vi "LoadControlPanel.vi"(8 "error in (no error)":errorcluster, 10 "Actor In":refnum<class "Actor.lvclass">, 11 "Laser_Oxxius in":refnum<class "Laser_Oxxius.lvclass">) -> (0 "error out":errorcluster, 3 "Laser_Oxxius out":refnum<class "Laser_Oxxius.lvclass">)   [LabVIEW 2020, in "Laser_Oxxius.lvlib" / "Laser_Oxxius.lvclass"]
uses:
  Laser_Oxxius.lvclass
  ViewController/OxxiusLaserController/OxxiusLaserController.lvclass
  Hardware Abstraction Layer/Component/Laser/Laser/Laser.lvclass
  C:/Program Files/National Instruments/LabVIEW 2020/vi.lib/ActorFramework/Actor/Actor.lvclass
  <vilib>/ActorFramework/Actor/Actor.lvclass
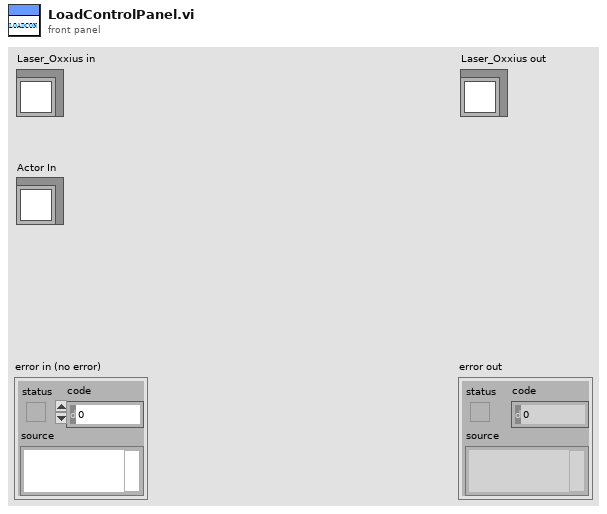
[diagram p1: front panel]
types:
  T1 = typedef "DataListener.lvclass/DataExchange.ctl" = cluster{"Source":string, "Destination":string, "Description":string, "value":variant}
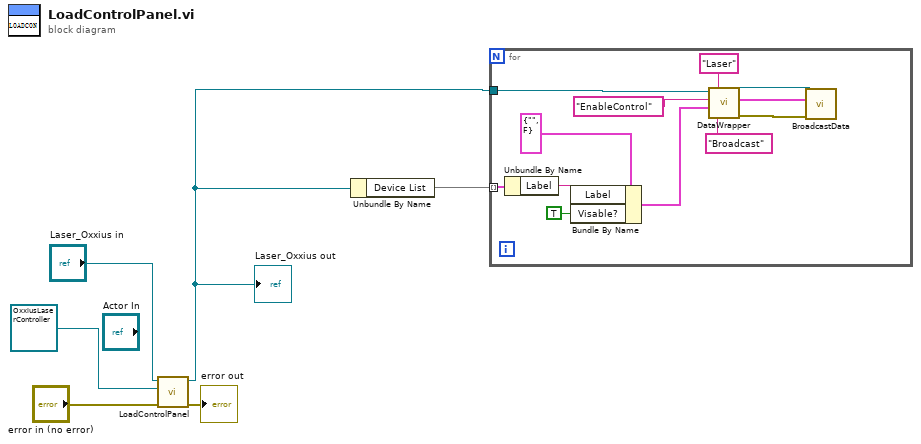
[diagram p0: block diagram]
diagram:
  n1 = call-parent "LoadControlPanel.vi"("error in (no error)"="error in (no error)", "Actor In"=refnum<class "OxxiusLaserController.lvclass"> refnum ("OxxiusLaserController.lvlib:OxxiusLaserController.lvclass"), "GRMActor in"="Laser_Oxxius in") -> ("error out"=→"error out":errorcluster, "GRMActor out"=w1:refnum<class "Laser_Oxxius.lvclass">)  [unwired: 7 in]
  "Laser_Oxxius out" <- w1
  n2 = Unbundle By Name(w1) -> ("Device List"=w2:map{string, refnum<k24>})
  n3 = for {
    tunnel: w2 -> [w18] mode=indexing
    tunnel: w1 -> [w14]
    n4 = Unbundle By Name(w18) -> ("Label"=w16:string)
    n5 = Bundle By Name(cluster=cluster{"Label":string, "Visable?":bool} {"Label"="", "Visable?"=FALSE} ("event data"), "Label"=w16, "Visable?"=TRUE) -> (w10:cluster{"Label":string, "Visable?":bool})
    n6 = call-dynamic "DataWrapper.vi"("Destination"="Broadcast" ("Type"), "Source"="Laser", "value"=w10, "Description"="EnableControl" ("Target"), "GRMActor in"=w14) -> ("error out"=w7:errorcluster, "DataExchange"=w8:T1, "GRMActor out"=w9:refnum<class "Laser_Oxxius.lvclass">)  [unwired: 4 in]
    n7 = call-dynamic "BroadcastData.vi"("error in (no error)"=w7, "DataExchange"=w8, "GRMActor in"=w9) -> ()  [unwired: 7 in, 2 out]
  }
